vi "INIT.vi"(8 "error in (no error)":errorcluster, 11 "USD ACTOR in":refnum<class "USD ACTOR.lvclass">) -> (0 "error out":errorcluster, 3 "USD ACTOR out":refnum<class "USD ACTOR.lvclass">)   [LabVIEW 2019, in "USD ACTOR.lvlib" / "USD ACTOR.lvclass"]
uses:
  USD ACTOR.lvclass
  USD ACTOR.lvclass/USD ACTOR.ctl
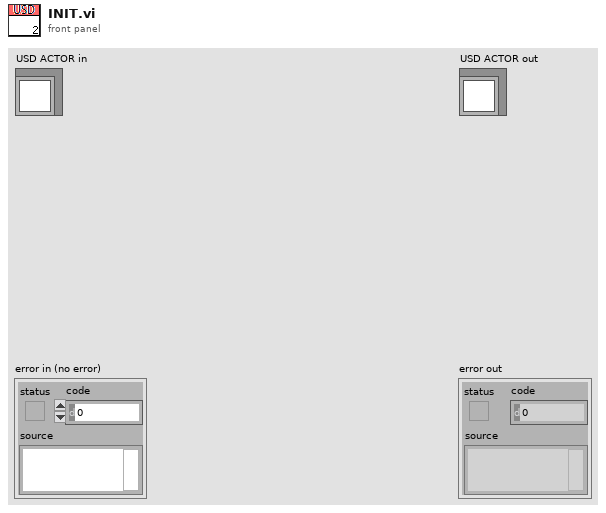
[diagram p1: front panel]
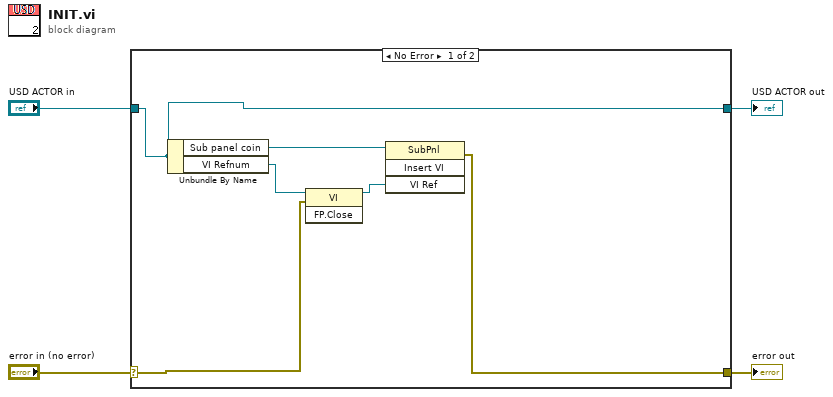
[diagram p0: block diagram]
diagram:
  n1 = case shown="No Error" "error in (no error)" {
    selector: "error in (no error)" -> [w6 w12]
    tunnel: [w5 w12] -> w3
    tunnel: [w10 w11] -> w1
    tunnel: "USD ACTOR in" -> [w10 w11]
    frame No Error {
      n2 = Unbundle By Name(w10) -> ("Sub panel coin"=w9:refnum<vi>, "VI Refnum"=w8:refnum<vi>)
      n3 = invoke class="VI" method="FP.Close"(reference=w8, error in=w6) -> (reference out=w7:refnum<vi>)  [unwired: 1 in, 2 out]
      n4 = invoke class="SubPnl" method="Insert VI"(reference=w9, "VI Ref"=w7) -> (error out=w5:errorcluster)  [unwired: 2 in, 3 out]
    }
    frame Error {
    }
  }
  "error out" <- w3
  "USD ACTOR out" <- w1
